vi "Pre Launch Init.vi"(11 "IMediator In":refnum<class "IMediator.lvclass">) -> (0 "error out":errorcluster, 3 "IMediator Out":refnum<class "IMediator.lvclass">)   [LabVIEW 2017, in "IMediator.lvlib" / "IMediator.lvclass"]
doc: "(<B>Filename</B>: Actor Framework.lvlib:Actor.lvclass:Pre Launch Init.vi)\n\nDefines behavior that occurs after the Launch Nested Actor method is invoked but before the actor's Actor Core method begins running.\n\nBy default, this method does nothing. A descendant class may override it to define behavior."
uses:
  IMediator.lvclass
  <vilib>/ActorFramework/Actor/Actor.lvclass
  gpm_packages/@cs/event-logger/Source/Composed Log/Types/Log Level.ctl
  gpm_packages/@cs/event-logger/Source/Composed Log/Composed Log.lvlib
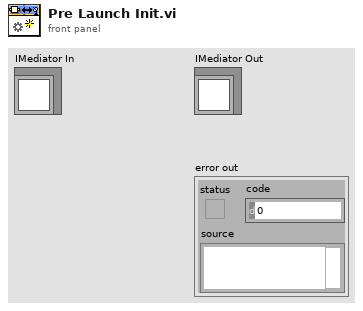
[diagram p1: front panel]
types:
  T1 = typedef "Composed Log.lvlib/Log Level.ctl" = enum16{"Debug", "Info", "Warning", "Error", "Critical"}
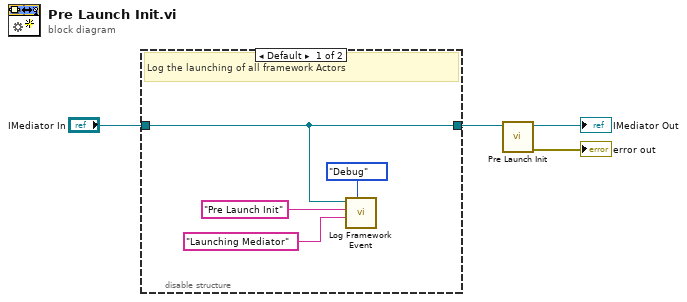
[diagram p0: block diagram]
diagram:
  n1 = disable-structure shown="Default" {
    disable-tunnel: "IMediator In" -> [w7 w9]
    disable-tunnel: [w7 w9] -> w2
    frame condition #0 (active) {
      # "Log the launching of all framework Actors"
      n2 = call "Log Framework Event.vi"("Event Level (Debug)"=Log_Level."Debug", "Data To Log"="Launching Mediator", "Caller Info (\"\")"="Pre Launch Init" ("Caller Info (\"\")"), "IMediator In"=w7) -> ()  [unwired: 7 in, 1 out]
    }
    frame condition #1 {
      # "Remove all logging from this method at compile time"
    }
  }
  n3 = call-parent "Pre Launch Init.vi"("Actor in"=w2) -> ("error out"=→"error out":errorcluster, "Actor out"=→"IMediator Out":refnum<class "IMediator.lvclass">)  [unwired: 9 in]
